vi "Post-Init.vi"(8 "error in (no error)":errorcluster, 11 "NI-Scope Lock-in Driver in":refnum<class "NI-Scope Lock-in Driver.lvclass">) -> (0 "error out":errorcluster, 2 "Init Result":refnum<class "Acquired Result.lvclass">, 3 "NI-Scope Lock-in Driver out":refnum<class "NI-Scope Lock-in Driver.lvclass">)   [LabVIEW 2016, in "NI-Scope Lock-in Driver.lvclass"]
uses:
  NI-Scope Lock-in Driver.lvclass
  C:/github/NHMFL_Core/Libraries/Instruments/Instrument Driver/Instrument Driver.lvclass
  Instruments/Results/Acquired Result/Acquired Result.lvclass
  Instruments/Instrument Driver/Instrument Driver.lvclass/Instrument Driver.ctl
  Instruments/Results/Acquired Result/Acquired Result.lvclass/Acquired Result.ctl
  Instruments/Instrument Driver/Read Channel names.vi
  Instruments/Instrument Driver/Write Channel names.vi
  Instruments/Instrument Driver/Write Channel units.vi
  Instruments/Results/Acquired Result/Write Channels.vi
  NI-Scope Digitizer/Ni-Scope Digitizer.lvclass
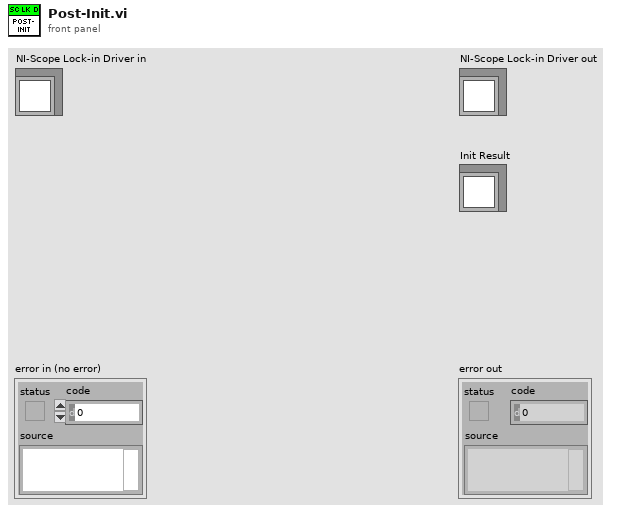
[diagram p1: front panel]
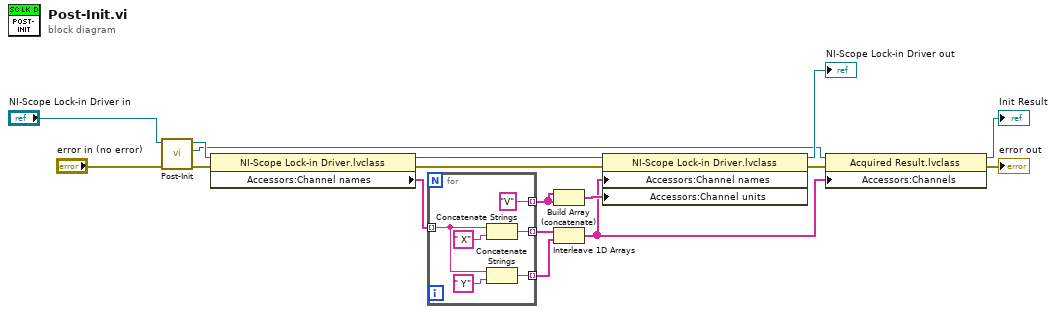
[diagram p0: block diagram]
diagram:
  n1 = call-parent "Post-Init.vi"("error in (no error)"="error in (no error)", "Pulse Driver in"="NI-Scope Lock-in Driver in") -> ("error out"=w17:errorcluster, "Init Result"=w5:refnum<class "Acquired Result.lvclass">, "Pulse Driver out"=w13:refnum<class "NI-Scope Lock-in Driver.lvclass">)  [unwired: 7 in]
  n2 = property class="NI-Scope Lock-in Driver.lvclass"(reference=w13, error in=w17) -> (reference out=w12:refnum<class "NI-Scope Lock-in Driver.lvclass">, error out=w14:errorcluster, "Accessors:Channel names"=w10:string[])
  n3 = for {
    tunnel: w10 -> [w22] mode=indexing
    tunnel: [w20] -> w9 mode=indexing
    tunnel: [w19] -> w8 mode=indexing
    tunnel: ["V" ("string")] -> w7 mode=indexing
    n4 = Concatenate Strings(w22, " X" ("string")) -> (w20:string)
    n5 = Concatenate Strings(w22, " Y" ("string")) -> (w19:string)
  }
  n6 = Build Array (concatenate)(w7, w7) -> (w6:string[])
  n7 = Interleave 1D Arrays(w9, w8) -> (w1:string[])
  n8 = property class="NI-Scope Lock-in Driver.lvclass"(reference=w12, error in=w14, "Accessors:Channel names"=w1, "Accessors:Channel units"=w6) -> (reference out=→"NI-Scope Lock-in Driver out":refnum<class "NI-Scope Lock-in Driver.lvclass">, error out=w3:errorcluster)
  n9 = property class="Acquired Result.lvclass"(reference=w5, error in=w3, "Accessors:Channels"=w1) -> (reference out=→"Init Result":refnum<class "Acquired Result.lvclass">, error out=→"error out":errorcluster)
